vi "Dresden Edit Recipe(in).vi"() -> ()   [LabVIEW 2009] (continued)
              }
              frame #25 {
                n1720 = local write "R Cmb Ch2 Target material"("Co" ("R DC Target material")) -> ()
              }
              frame #26 {
                n1721 = local write "R Cmb Ch2 Target material"("Cu" ("R DC Target material")) -> ()
              }
              frame #27 {
                n1722 = local write "R Cmb Ch2 Target material"("Cu2S (A)" ("R DC Target material")) -> ()
              }
              frame #28 {
                n1723 = local write "R Cmb Ch2 Target material"("Cu2S (B)" ("R DC Target material")) -> ()
              }
              frame #29 {
                n1724 = local write "R Cmb Ch2 Target material"("CuS" ("R DC Target material")) -> ()
              }
              frame #30 {
                n1725 = local write "R Cmb Ch2 Target material"("Dy" ("R DC Target material")) -> ()
              }
              frame #31 {
                n1726 = local write "R Cmb Ch2 Target material"("Er" ("R DC Target material")) -> ()
              }
              frame #32 {
                n1727 = local write "R Cmb Ch2 Target material"("Fe" ("R DC Target material")) -> ()
              }
              frame #33 {
                n1728 = local write "R Cmb Ch2 Target material"("Ga" ("R DC Target material")) -> ()
              }
              frame #34 {
                n1729 = local write "R Cmb Ch2 Target material"("GaAs" ("R DC Target material")) -> ()
              }
              frame #35 {
                n1730 = local write "R Cmb Ch2 Target material"("Gd" ("R DC Target material")) -> ()
              }
              frame #36 {
                n1731 = local write "R Cmb Ch2 Target material"("Ge" ("R DC Target material")) -> ()
              }
              frame #37 {
                n1732 = local write "R Cmb Ch2 Target material"("Hf" ("R DC Target material")) -> ()
              }
              frame #38 {
                n1733 = local write "R Cmb Ch2 Target material"("HfO2" ("R DC Target material")) -> ()
              }
              frame #39 {
                n1734 = local write "R Cmb Ch2 Target material"("Hg" ("R DC Target material")) -> ()
              }
              frame #40 {
                n1735 = local write "R Cmb Ch2 Target material"("Ho" ("R DC Target material")) -> ()
              }
              frame #41 {
                n1736 = local write "R Cmb Ch2 Target material"("In" ("R DC Target material")) -> ()
              }
              frame #42 {
                n1737 = local write "R Cmb Ch2 Target material"("InSb" ("R DC Target material")) -> ()
              }
              frame #43 {
                n1738 = local write "R Cmb Ch2 Target material"("In2O3" ("R DC Target material")) -> ()
              }
              frame #44 {
                n1739 = local write "R Cmb Ch2 Target material"("Ir" ("R DC Target material")) -> ()
              }
              frame #45 {
                n1740 = local write "R Cmb Ch2 Target material"("KCl" ("R DC Target material")) -> ()
              }
              frame #46 {
                n1741 = local write "R Cmb Ch2 Target material"("La" ("R DC Target material")) -> ()
              }
              frame #47 {
                n1742 = local write "R Cmb Ch2 Target material"("LaF3" ("R DC Target material")) -> ()
              }
              frame #48 {
                n1743 = local write "R Cmb Ch2 Target material"("LaO3" ("R DC Target material")) -> ()
              }
              frame #49 {
                n1744 = local write "R Cmb Ch2 Target material"("Li" ("R DC Target material")) -> ()
              }
              frame #50 {
                n1745 = local write "R Cmb Ch2 Target material"("LiF" ("R DC Target material")) -> ()
              }
              frame #51 {
                n1746 = local write "R Cmb Ch2 Target material"("Mg" ("R DC Target material")) -> ()
              }
              frame #52 {
                n1747 = local write "R Cmb Ch2 Target material"("MgF2" ("R DC Target material")) -> ()
              }
              frame #53 {
                n1748 = local write "R Cmb Ch2 Target material"("MgO" ("R DC Target material")) -> ()
              }
              frame #54 {
                n1749 = local write "R Cmb Ch2 Target material"("Mn" ("R DC Target material")) -> ()
              }
              frame #55 {
                n1750 = local write "R Cmb Ch2 Target material"("MnS" ("R DC Target material")) -> ()
              }
              frame #56 {
                n1751 = local write "R Cmb Ch2 Target material"("Mo" ("R DC Target material")) -> ()
              }
              frame #57 {
                n1752 = local write "R Cmb Ch2 Target material"("Na" ("R DC Target material")) -> ()
              }
              frame #58 {
                n1753 = local write "R Cmb Ch2 Target material"("NaCl" ("R DC Target material")) -> ()
              }
              frame #59 {
                n1754 = local write "R Cmb Ch2 Target material"("NdF3" ("R DC Target material")) -> ()
              }
              frame #60 {
                n1755 = local write "R Cmb Ch2 Target material"("Nd2O3" ("R DC Target material")) -> ()
              }
              frame #61 {
                n1756 = local write "R Cmb Ch2 Target material"("Ni" ("R DC Target material")) -> ()
              }
              frame #62 {
                n1757 = local write "R Cmb Ch2 Target material"("Nb" ("R DC Target material")) -> ()
              }
              frame #63 {
                n1758 = local write "R Cmb Ch2 Target material"("Nb2O5" ("R DC Target material")) -> ()
              }
              frame #64 {
                n1759 = local write "R Cmb Ch2 Target material"("Pb" ("R DC Target material")) -> ()
              }
              frame #65 {
                n1760 = local write "R Cmb Ch2 Target material"("PbS" ("R DC Target material")) -> ()
              }
              frame #66 {
                n1761 = local write "R Cmb Ch2 Target material"("Pd" ("R DC Target material")) -> ()
              }
              frame #67 {
                n1762 = local write "R Cmb Ch2 Target material"("Pt" ("R DC Target material")) -> ()
              }
              frame #68 {
                n1763 = local write "R Cmb Ch2 Target material"("Re" ("R DC Target material")) -> ()
              }
              frame #69 {
                n1764 = local write "R Cmb Ch2 Target material"("Rh" ("R DC Target material")) -> ()
              }
              frame #70 {
                n1765 = local write "R Cmb Ch2 Target material"("Rb" ("R DC Target material")) -> ()
              }
              frame #71 {
                n1766 = local write "R Cmb Ch2 Target material"("S" ("R DC Target material")) -> ()
              }
              frame #72 {
                n1767 = local write "R Cmb Ch2 Target material"("Sb" ("R DC Target material")) -> ()
              }
              frame #73 {
                n1768 = local write "R Cmb Ch2 Target material"("Sc" ("R DC Target material")) -> ()
              }
              frame #74 {
                n1769 = local write "R Cmb Ch2 Target material"("Se" ("R DC Target material")) -> ()
              }
              frame #75 {
                n1770 = local write "R Cmb Ch2 Target material"("Si" ("R DC Target material")) -> ()
              }
              frame #76 {
                n1771 = local write "R Cmb Ch2 Target material"("SiO" ("R DC Target material")) -> ()
              }
              frame #77 {
                n1772 = local write "R Cmb Ch2 Target material"("SiO2" ("R DC Target material")) -> ()
              }
              frame #78 {
                n1773 = local write "R Cmb Ch2 Target material"("Sm" ("R DC Target material")) -> ()
              }
              frame #79 {
                n1774 = local write "R Cmb Ch2 Target material"("Sn" ("R DC Target material")) -> ()
              }
              frame #80 {
                n1775 = local write "R Cmb Ch2 Target material"("Ta" ("R DC Target material")) -> ()
              }
              frame #81 {
                n1776 = local write "R Cmb Ch2 Target material"("Ta2O5" ("R DC Target material")) -> ()
              }
              frame #82 {
                n1777 = local write "R Cmb Ch2 Target material"("Te" ("R DC Target material")) -> ()
              }
              frame #83 {
                n1778 = local write "R Cmb Ch2 Target material"("Tb" ("R DC Target material")) -> ()
              }
              frame #84 {
                n1779 = local write "R Cmb Ch2 Target material"("ThF4" ("R DC Target material")) -> ()
              }
              frame #85 {
                n1780 = local write "R Cmb Ch2 Target material"("Ti" ("R DC Target material")) -> ()
              }
              frame #86 {
                n1781 = local write "R Cmb Ch2 Target material"("TiO2" ("R DC Target material")) -> ()
              }
              frame #87 {
                n1782 = local write "R Cmb Ch2 Target material"("TiO" ("R DC Target material")) -> ()
              }
              frame #88 {
                n1783 = local write "R Cmb Ch2 Target material"("Tl" ("R DC Target material")) -> ()
              }
              frame #89 {
                n1784 = local write "R Cmb Ch2 Target material"("U" ("R DC Target material")) -> ()
              }
              frame #90 {
                n1785 = local write "R Cmb Ch2 Target material"("V" ("R DC Target material")) -> ()
              }
              frame #91 {
                n1786 = local write "R Cmb Ch2 Target material"("W" ("R DC Target material")) -> ()
              }
              frame #92 {
                n1787 = local write "R Cmb Ch2 Target material"("WC" ("R DC Target material")) -> ()
              }
              frame #93 {
                n1788 = local write "R Cmb Ch2 Target material"("Y" ("R DC Target material")) -> ()
              }
              frame #94 {
                n1789 = local write "R Cmb Ch2 Target material"("Y2O3" ("R DC Target material")) -> ()
              }
              frame #95 {
                n1790 = local write "R Cmb Ch2 Target material"("Yb" ("R DC Target material")) -> ()
              }
              frame #96 {
                n1791 = local write "R Cmb Ch2 Target material"("Zn" ("R DC Target material")) -> ()
              }
              frame #97 {
                n1792 = local write "R Cmb Ch2 Target material"("ZnO" ("R DC Target material")) -> ()
              }
              frame #98 {
                n1793 = local write "R Cmb Ch2 Target material"("ZnSe" ("R DC Target material")) -> ()
              }
              frame #99 {
                n1794 = local write "R Cmb Ch2 Target material"("ZnS" ("R DC Target material")) -> ()
              }
              frame #100 {
                n1795 = local write "R Cmb Ch2 Target material"("Zr" ("R DC Target material")) -> ()
              }
              frame #101 {
                n1796 = local write "R Cmb Ch2 Target material"("ZrO2" ("R DC Target material")) -> ()
              }
              frame #102 {
                n1797 = local write "R Cmb Ch2 Target material"("Si3N4" ("R DC Target material")) -> ()
              }
              frame #103 {
                n1798 = local write "R Cmb Ch2 Target material"("ITO" ("R DC Target material")) -> ()
              }
              frame #104 {
                n1799 = local write "R Cmb Ch2 Target material"("PbI2" ("R DC Target material")) -> ()
              }
            }
            n1800 = local read "Web_selection_tab"() -> (w1009:T4)
            n1801 = case shown="\"Multilayer Recipe                                                                  \"" w986 {
              frame #0 {
              }
              frame #1 {
                n1802 = local write "R_Simple_Coating Type Selection"(T2."DC Sputter" ("R_Simple_Coating Type Selection")) -> ()
              }
            }
            n1803 = local read "R Single RF Step8 Coating Power Active"() -> (w833:bool)
            n1804 = case shown="True" w832 {
              frame #0 {
              }
              frame #1 {
                n1805 = local read "R Cmb Step2 Coating Power Active"() -> (w1069:bool)
                n1806 = case shown="False" w1069 {
                  frame #0 {
                    w1070 = 0.0 ("R Cmb Ch2 Step2 Coating Power")
                    w1071 = T5."Disabled and Grayed Out" ("Disabled")
                    n1807 = local write "R Cmb Ch3 Step2 Coating Power"(w1070) -> ()
                    n1808 = local write "R Cmb Ch2 Step2 Coating Power"(w1070) -> ()
                    n1809 = local write "R Cmb Interval length 2"(w1070) -> ()
                    n1810 = property on="R Cmb Ch2 Step2 Coating Power" class="DigNum (strict)"("DisabledEnum"=w1071) -> ()  [unwired: 2 in, 2 out]
                    n1811 = property on="R Cmb Ch3 Step2 Coating Power" class="DigNum (strict)"("DisabledEnum"=w1071) -> ()  [unwired: 2 in, 2 out]
                    n1812 = property on="R Cmb Interval length 2" class="DigNum (strict)"("DisabledEnum"=w1071) -> ()  [unwired: 2 in, 2 out]
                  }
                  frame #1 {
                    w1072 = T5."Enabled" ("Disabled")
                    n1813 = property on="R Cmb Ch2 Step2 Coating Power" class="DigNum (strict)"("DisabledEnum"=w1072) -> ()  [unwired: 2 in, 2 out]
                    n1814 = property on="R Cmb Ch3 Step2 Coating Power" class="DigNum (strict)"("DisabledEnum"=w1072) -> ()  [unwired: 2 in, 2 out]
                    n1815 = property on="R Cmb Interval length 2" class="DigNum (strict)"("DisabledEnum"=w1072) -> ()  [unwired: 2 in, 2 out]
                  }
                }
              }
            }
            n1816 = case shown="True" w831 {
              frame #0 {
                w1064 = FALSE ("R Cmb Step3 Coating Power Active")
                n1817 = local write "R Cmb Step3 Coating Power Active"(w1064) -> ()
                n1818 = local write "R Cmb Step4 Coating Power Active"(w1064) -> ()
                n1819 = local write "R Cmb Step5 Coating Power Active"(w1064) -> ()
                n1820 = local write "R Cmb Step6 Coating Power Active"(w1064) -> ()
                n1821 = local write "R Cmb Step7 Coating Power Active"(w1064) -> ()
                n1822 = local write "R Cmb Step8 Coating Power Active"(w1064) -> ()
                n1823 = local write "R Cmb Step9 Coating Power Active"(w1064) -> ()
                n1824 = local write "R Cmb Step10 Coating Power Active"(w1064) -> ()
              }
              frame #1 {
                n1825 = local read "R Cmb Step3 Coating Power Active"() -> (w1065:bool)
                n1826 = case shown="False" w1065 {
                  frame #0 {
                    w1066 = 0.0 ("R Cmb Ch2 Step3 Coating Power")
                    w1067 = T5."Disabled and Grayed Out" ("Disabled")
                    n1827 = local write "R Cmb Ch2 Step3 Coating Power"(w1066) -> ()
                    n1828 = local write "R Cmb Ch3 Step3 Coating Power"(w1066) -> ()
                    n1829 = local write "R Cmb Interval length 3"(w1066) -> ()
                    n1830 = property on="R Cmb Ch3 Step3 Coating Power" class="DigNum (strict)"("DisabledEnum"=w1067) -> ()  [unwired: 2 in, 2 out]
                    n1831 = property on="R Cmb Interval length 3" class="DigNum (strict)"("DisabledEnum"=w1067) -> ()  [unwired: 2 in, 2 out]
                    n1832 = property on="R Cmb Ch2 Step3 Coating Power" class="DigNum (strict)"("DisabledEnum"=w1067) -> ()  [unwired: 2 in, 2 out]
                  }
                  frame #1 {
                    w1068 = T5."Enabled" ("Disabled")
                    n1833 = property on="R Cmb Ch3 Step3 Coating Power" class="DigNum (strict)"("DisabledEnum"=w1068) -> ()  [unwired: 2 in, 2 out]
                    n1834 = property on="R Cmb Interval length 3" class="DigNum (strict)"("DisabledEnum"=w1068) -> ()  [unwired: 2 in, 2 out]
                    n1835 = property on="R Cmb Ch2 Step3 Coating Power" class="DigNum (strict)"("DisabledEnum"=w1068) -> ()  [unwired: 2 in, 2 out]
                  }
                }
              }
            }
            n1836 = case shown="False" w829 {
              frame #0 {
                w1054 = FALSE ("R Cmb Step3 Coating Power Active")
                n1837 = local write "R Cmb Step5 Coating Power Active"(w1054) -> ()
                n1838 = local write "R Cmb Step6 Coating Power Active"(w1054) -> ()
                n1839 = local write "R Cmb Step7 Coating Power Active"(w1054) -> ()
                n1840 = local write "R Cmb Step8 Coating Power Active"(w1054) -> ()
                n1841 = local write "R Cmb Step9 Coating Power Active"(w1054) -> ()
                n1842 = local write "R Cmb Step10 Coating Power Active"(w1054) -> ()
              }
              frame #1 {
                n1843 = local read "R Cmb Step5 Coating Power Active"() -> (w1055:bool)
                n1844 = case shown="False" w1055 {
                  frame #0 {
                    w1056 = 0.0 ("R Cmb Ch2 Step5 Coating Power")
                    w1057 = T5."Disabled and Grayed Out" ("Disabled")
                    n1845 = local write "R Cmb Ch2 Step5 Coating Power"(w1056) -> ()
                    n1846 = local write "R Cmb Ch3 Step5 Coating Power"(w1056) -> ()
                    n1847 = local write "R Cmb Interval length 5"(w1056) -> ()
                    n1848 = property on="R Cmb Ch3 Step5 Coating Power" class="DigNum (strict)"("DisabledEnum"=w1057) -> ()  [unwired: 2 in, 2 out]
                    n1849 = property on="R Cmb Interval length 5" class="DigNum (strict)"("DisabledEnum"=w1057) -> ()  [unwired: 2 in, 2 out]
                    n1850 = property on="R Cmb Ch2 Step5 Coating Power" class="DigNum (strict)"("DisabledEnum"=w1057) -> ()  [unwired: 2 in, 2 out]
                  }
                  frame #1 {
                    w1058 = T5."Enabled" ("Disabled")
                    n1851 = property on="R Cmb Ch3 Step5 Coating Power" class="DigNum (strict)"("DisabledEnum"=w1058) -> ()  [unwired: 2 in, 2 out]
                    n1852 = property on="R Cmb Interval length 5" class="DigNum (strict)"("DisabledEnum"=w1058) -> ()  [unwired: 2 in, 2 out]
                    n1853 = property on="R Cmb Ch2 Step5 Coating Power" class="DigNum (strict)"("DisabledEnum"=w1058) -> ()  [unwired: 2 in, 2 out]
                  }
                }
              }
            }
            n1854 = case shown="True" w830 {
              frame #0 {
                w1059 = FALSE ("R Cmb Step3 Coating Power Active")
                n1855 = local write "R Cmb Step4 Coating Power Active"(w1059) -> ()
                n1856 = local write "R Cmb Step5 Coating Power Active"(w1059) -> ()
                n1857 = local write "R Cmb Step6 Coating Power Active"(w1059) -> ()
                n1858 = local write "R Cmb Step7 Coating Power Active"(w1059) -> ()
                n1859 = local write "R Cmb Step8 Coating Power Active"(w1059) -> ()
                n1860 = local write "R Cmb Step9 Coating Power Active"(w1059) -> ()
                n1861 = local write "R Cmb Step10 Coating Power Active"(w1059) -> ()
              }
              frame #1 {
                n1862 = local read "R Cmb Step4 Coating Power Active"() -> (w1060:bool)
                n1863 = case shown="False" w1060 {
                  frame #0 {
                    w1061 = 0.0 ("R Cmb Ch2 Step4 Coating Power")
                    w1062 = T5."Disabled and Grayed Out" ("Disabled")
                    n1864 = local write "R Cmb Ch2 Step4 Coating Power"(w1061) -> ()
                    n1865 = local write "R Cmb Ch3 Step4 Coating Power"(w1061) -> ()
                    n1866 = local write "R Cmb Interval length 4"(w1061) -> ()
                    n1867 = property on="R Cmb Ch2 Step4 Coating Power" class="DigNum (strict)"("DisabledEnum"=w1062) -> ()  [unwired: 2 in, 2 out]
                    n1868 = property on="R Cmb Ch3 Step4 Coating Power" class="DigNum (strict)"("DisabledEnum"=w1062) -> ()  [unwired: 2 in, 2 out]
                    n1869 = property on="R Cmb Interval length 4" class="DigNum (strict)"("DisabledEnum"=w1062) -> ()  [unwired: 2 in, 2 out]
                  }
                  frame #1 {
                    w1063 = T5."Enabled" ("Disabled")
                    n1870 = property on="R Cmb Ch2 Step4 Coating Power" class="DigNum (strict)"("DisabledEnum"=w1063) -> ()  [unwired: 2 in, 2 out]
                    n1871 = property on="R Cmb Ch3 Step4 Coating Power" class="DigNum (strict)"("DisabledEnum"=w1063) -> ()  [unwired: 2 in, 2 out]
                    n1872 = property on="R Cmb Interval length 4" class="DigNum (strict)"("DisabledEnum"=w1063) -> ()  [unwired: 2 in, 2 out]
                  }
                }
              }
            }
            n1873 = local read "R Cmb Step1 Coating Power Active"() -> (w984:bool)
            n1874 = case shown="True" "Power_singledc_list_open" {
              frame #0 {
                n1875 = property on="Single_DC_power_power_tab" class="TabCtl (strict)"("Visible"=FALSE) -> ()  [unwired: 2 in, 2 out]
              }
              frame #1 {
                n1876 = property on="Single_DC_power_power_tab" class="TabCtl (strict)"("Visible"=TRUE) -> ()  [unwired: 2 in, 2 out]
              }
            }
            n1877 = Equal?(x=w1009, y=1) -> (x = y?=w1007:bool)
            n1878 = case shown="True" w1007 {
              frame #0 {
                n1879 = property on="R_Single Microwave Time" class="DigNum (strict)"("DisabledEnum"=T5."Disabled and Grayed Out" ("Disabled")) -> ()  [unwired: 2 in, 2 out]
              }
              frame #1 {
                w2483 = 0.0 ("R Single DC Step2 Coating Power")
                w2481 = T5."Disabled and Grayed Out" ("Disabled")
                w2482 = FALSE ("R Single DC Step2 Coating Power Active")
                n1880 = local write "R Single RF Step2 Coating Power Active"(w2482) -> ()
                n1881 = local write "R Single RF Step3 Coating Power Active"(w2482) -> ()
                n1882 = local write "R Single RF Step4 Coating Power Active"(w2482) -> ()
                n1883 = local write "R Single RF Step5 Coating Power Active"(w2482) -> ()
                n1884 = local write "R Single RF Step6 Coating Power Active"(w2482) -> ()
                n1885 = local write "R Single RF Step7 Coating Power Active"(w2482) -> ()
                n1886 = local write "R Single RF Step8 Coating Power Active"(w2482) -> ()
                n1887 = local write "R Single RF Step9 Coating Power Active"(w2482) -> ()
                n1888 = local write "R Single RF Step10 Coating Power Active"(w2482) -> ()
                n1889 = local write "R Single DC Step2 Coating Power Active"(w2482) -> ()
                n1890 = local write "R Single DC Step3 Coating Power Active"(w2482) -> ()
                n1891 = local write "R Single DC Step4 Coating Power Active"(w2482) -> ()
                n1892 = local write "R Single DC Step5 Coating Power Active"(w2482) -> ()
                n1893 = local write "R Single DC Step6 Coating Power Active"(w2482) -> ()
                n1894 = local write "R Single DC Step7 Coating Power Active"(w2482) -> ()
                n1895 = local write "R Single DC Step8 Coating Power Active"(w2482) -> ()
                n1896 = local write "R Single DC Step9 Coating Power Active"(w2482) -> ()
                n1897 = local write "R Single DC Step10 Coating Power Active"(w2482) -> ()
                n1898 = local write "R Single DC Step2 Coating Power"(w2483) -> ()
                n1899 = local write "R Single DC Step3 Coating Power"(w2483) -> ()
                n1900 = local write "R Single DC Step4 Coating Power"(w2483) -> ()
                n1901 = local write "R Single DC Step5 Coating Power"(w2483) -> ()
                n1902 = local write "R Single RF Step2 Coating Power"(w2483) -> ()
                n1903 = local write "R Single RF Step3 Coating Power"(w2483) -> ()
                n1904 = local write "R Single RF Step4 Coating Power"(w2483) -> ()
                n1905 = local write "R Single RF Step5 Coating Power"(w2483) -> ()
                n1906 = local write "R Single DC Step6 Coating Power"(w2483) -> ()
                n1907 = local write "R Single DC Step7 Coating Power"(w2483) -> ()
                n1908 = local write "R Single DC Step8 Coating Power"(w2483) -> ()
                n1909 = local write "R Single DC Step9 Coating Power"(w2483) -> ()
                n1910 = local write "R Single DC Step10 Coating Power"(w2483) -> ()
                n1911 = local write "R Single RF Step6 Coating Power"(w2483) -> ()
                n1912 = local write "R Single RF Step7 Coating Power"(w2483) -> ()
                n1913 = local write "R Single RF Step8 Coating Power"(w2483) -> ()
                n1914 = local write "R Single RF Step9 Coating Power"(w2483) -> ()
                n1915 = local write "R Single RF Step10 Coating Power"(w2483) -> ()
                n1916 = property on="R_Single Microwave Time" class="DigNum (strict)"("DisabledEnum"=T5."Enabled" ("Disabled")) -> ()  [unwired: 2 in, 2 out]
                n1917 = property on="R Single DC Step2 Coating Power" class="DigNum (strict)"("DisabledEnum"=w2481) -> ()  [unwired: 2 in, 2 out]
                n1918 = property on="R Single DC Step3 Coating Power" class="DigNum (strict)"("DisabledEnum"=w2481) -> ()  [unwired: 2 in, 2 out]
                n1919 = property on="R Single DC Step4 Coating Power" class="DigNum (strict)"("DisabledEnum"=w2481) -> ()  [unwired: 2 in, 2 out]
                n1920 = property on="R Single DC Step5 Coating Power" class="DigNum (strict)"("DisabledEnum"=w2481) -> ()  [unwired: 2 in, 2 out]
                n1921 = property on="R Single RF Step2 Coating Power" class="DigNum (strict)"("DisabledEnum"=w2481) -> ()  [unwired: 2 in, 2 out]
                n1922 = property on="R Single RF Step3 Coating Power" class="DigNum (strict)"("DisabledEnum"=w2481) -> ()  [unwired: 2 in, 2 out]
                n1923 = property on="R Single RF Step4 Coating Power" class="DigNum (strict)"("DisabledEnum"=w2481) -> ()  [unwired: 2 in, 2 out]
                n1924 = property on="R Single RF Step5 Coating Power" class="DigNum (strict)"("DisabledEnum"=w2481) -> ()  [unwired: 2 in, 2 out]
                n1925 = property on="R Single RF Step6 Coating Power" class="DigNum (strict)"("DisabledEnum"=w2481) -> ()  [unwired: 2 in, 2 out]
                n1926 = property on="R Single RF Step7 Coating Power" class="DigNum (strict)"("DisabledEnum"=w2481) -> ()  [unwired: 2 in, 2 out]
                n1927 = property on="R Single RF Step8 Coating Power" class="DigNum (strict)"("DisabledEnum"=w2481) -> ()  [unwired: 2 in, 2 out]
                n1928 = property on="R Single RF Step9 Coating Power" class="DigNum (strict)"("DisabledEnum"=w2481) -> ()  [unwired: 2 in, 2 out]
                n1929 = property on="R Single RF Step10 Coating Power" class="DigNum (strict)"("DisabledEnum"=w2481) -> ()  [unwired: 2 in, 2 out]
                n1930 = local write "R Single DC Interval length2"(w2483) -> ()
                n1931 = local write "R Single DC Interval length3"(w2483) -> ()
                n1932 = local write "R Single DC Interval length4"(w2483) -> ()
                n1933 = local write "R Single DC Interval length5"(w2483) -> ()
                n1934 = local write "R Single DC Interval length6"(w2483) -> ()
                n1935 = local write "R Single DC Interval length7"(w2483) -> ()
                n1936 = local write "R Single DC Interval length8"(w2483) -> ()
                n1937 = local write "R Single DC Interval length9"(w2483) -> ()
                n1938 = local write "R Single DC Interval length10"(w2483) -> ()
                n1939 = local write "R Single RF Interval length2"(w2483) -> ()
                n1940 = local write "R Single RF Interval length3"(w2483) -> ()
                n1941 = local write "R Single RF Interval length4"(w2483) -> ()
                n1942 = local write "R Single RF Interval length5"(w2483) -> ()
                n1943 = local write "R Single RF Interval length6"(w2483) -> ()
                n1944 = local write "R Single RF Interval length7"(w2483) -> ()
                n1945 = local write "R Single RF Interval length8"(w2483) -> ()
                n1946 = local write "R Single RF Interval length9"(w2483) -> ()
                n1947 = local write "R Single RF Interval length10"(w2483) -> ()
                n1948 = property on="R Single DC Interval length6" class="DigNum (strict)"("DisabledEnum"=w2481) -> ()  [unwired: 2 in, 2 out]
                n1949 = property on="R Single DC Interval length7" class="DigNum (strict)"("DisabledEnum"=w2481) -> ()  [unwired: 2 in, 2 out]
                n1950 = property on="R Single DC Interval length8" class="DigNum (strict)"("DisabledEnum"=w2481) -> ()  [unwired: 2 in, 2 out]
                n1951 = property on="R Single DC Interval length9" class="DigNum (strict)"("DisabledEnum"=w2481) -> ()  [unwired: 2 in, 2 out]
                n1952 = property on="R Single DC Interval length10" class="DigNum (strict)"("DisabledEnum"=w2481) -> ()  [unwired: 2 in, 2 out]
                n1953 = property on="R Single RF Interval length2" class="DigNum (strict)"("DisabledEnum"=w2481) -> ()  [unwired: 2 in, 2 out]
                n1954 = property on="R Single RF Interval length3" class="DigNum (strict)"("DisabledEnum"=w2481) -> ()  [unwired: 2 in, 2 out]
                n1955 = property on="R Single RF Interval length4" class="DigNum (strict)"("DisabledEnum"=w2481) -> ()  [unwired: 2 in, 2 out]
                n1956 = property on="R Single RF Interval length5" class="DigNum (strict)"("DisabledEnum"=w2481) -> ()  [unwired: 2 in, 2 out]
                n1957 = property on="R Single RF Interval length6" class="DigNum (strict)"("DisabledEnum"=w2481) -> ()  [unwired: 2 in, 2 out]
                n1958 = property on="R Single RF Interval length7" class="DigNum (strict)"("DisabledEnum"=w2481) -> ()  [unwired: 2 in, 2 out]
                n1959 = property on="R Single RF Interval length8" class="DigNum (strict)"("DisabledEnum"=w2481) -> ()  [unwired: 2 in, 2 out]
                n1960 = property on="R Single RF Interval length9" class="DigNum (strict)"("DisabledEnum"=w2481) -> ()  [unwired: 2 in, 2 out]
                n1961 = property on="R Single RF Interval length10" class="DigNum (strict)"("DisabledEnum"=w2481) -> ()  [unwired: 2 in, 2 out]
                n1962 = property on="R Single DC Step6 Coating Power" class="DigNum (strict)"("DisabledEnum"=w2481) -> ()  [unwired: 2 in, 2 out]
                n1963 = property on="R Single DC Step7 Coating Power" class="DigNum (strict)"("DisabledEnum"=w2481) -> ()  [unwired: 2 in, 2 out]
                n1964 = property on="R Single DC Step8 Coating Power" class="DigNum (strict)"("DisabledEnum"=w2481) -> ()  [unwired: 2 in, 2 out]
                n1965 = property on="R Single DC Step9 Coating Power" class="DigNum (strict)"("DisabledEnum"=w2481) -> ()  [unwired: 2 in, 2 out]
                n1966 = property on="R Single DC Step10 Coating Power" class="DigNum (strict)"("DisabledEnum"=w2481) -> ()  [unwired: 2 in, 2 out]
                n1967 = property on="R Single DC Interval length2" class="DigNum (strict)"("DisabledEnum"=w2481) -> ()  [unwired: 2 in, 2 out]
                n1968 = property on="R Single DC Interval length3" class="DigNum (strict)"("DisabledEnum"=w2481) -> ()  [unwired: 2 in, 2 out]
                n1969 = property on="R Single DC Interval length4" class="DigNum (strict)"("DisabledEnum"=w2481) -> ()  [unwired: 2 in, 2 out]
                n1970 = property on="R Single DC Interval length5" class="DigNum (strict)"("DisabledEnum"=w2481) -> ()  [unwired: 2 in, 2 out]
              }
            }
            n1971 = case shown="False" w833 {
              frame #0 {
                w1073 = FALSE ("R Single RF Step3 Coating Power Active")
                n1972 = local write "R Single RF Step9 Coating Power Active"(w1073) -> ()
                n1973 = local write "R Single RF Step10 Coating Power Active"(w1073) -> ()
              }
              frame #1 {
                n1974 = local read "R Single RF Step9 Coating Power Active"() -> (w1074:bool)
                n1975 = case shown="False" w1074 {
                  frame #0 {
                    w1075 = 0.0 ("Target Clean Power")
                    w1076 = T5."Disabled and Grayed Out" ("Disabled")
                    n1976 = local write "R Single RF Step9 Coating Power"(w1075) -> ()
                    n1977 = local write "R Single RF Interval length9"(w1075) -> ()
                    n1978 = property on="R Single RF Step9 Coating Power" class="DigNum (strict)"("DisabledEnum"=w1076) -> ()  [unwired: 2 in, 2 out]
                    n1979 = property on="R Single RF Interval length9" class="DigNum (strict)"("DisabledEnum"=w1076) -> ()  [unwired: 2 in, 2 out]
                  }
                  frame #1 {
                    w1077 = T5."Enabled" ("Disabled")
                    n1980 = property on="R Single RF Step9 Coating Power" class="DigNum (strict)"("DisabledEnum"=w1077) -> ()  [unwired: 2 in, 2 out]
